vi "background worker.vi"(11 "connection server in":refnum<class "connection server.lvclass">) -> ()   [LabVIEW 2015, in "connection server.lvclass"]
uses:
  connection server.lvclass
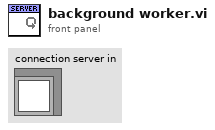
[diagram p1: front panel]
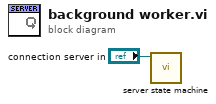
[diagram p0: block diagram]
diagram:
  n1 = call "server state machine.vi"("connection server in"="connection server in") -> ()  [unwired: 11 in]
